vi "tes2-testModuleTurnsInvalidAPI.vi"(8 "error in (no error)":errorcluster, 11 "TestCase in":refnum<class "testcase-CSMNonCSMCallerSupportAPI.lvclass">) -> (0 "error out":errorcluster, 3 "TestCase out":refnum<class "testcase-CSMNonCSMCallerSupportAPI.lvclass">)   [LabVIEW 2017, in "testcase-CSMNonCSMCallerSupportAPI.lvclass"]
uses:
  testcase-CSMNonCSMCallerSupportAPI.lvclass
  <vilib>/addons/_JKI Toolkits/VI Tester/TestCase.llb/TestCase.lvclass
  src/user.lib/_NEVSTOP/Communicable State Machine(CSM)/Communicable State Machine.lvlib
  src/user.lib/_NEVSTOP/Communicable State Machine(CSM)/_Support/Typedef/_CSM_List Module Scope.ctl
  GlobalVariable_CSMModeData.vi
  InternalCluster.ctl
  C:/Program Files (x86)/National Instruments/LabVIEW 2017/vi.lib/addons/_JKI Toolkits/VI Tester/TestCase.llb/TestCase.lvclass
panel:
  in  "Stop":bool
  out "error out 2":errorcluster
  out "LoopCount":i32
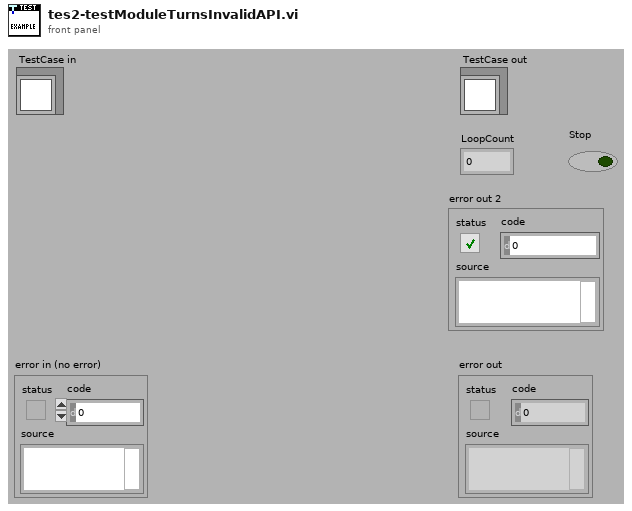
[diagram p1: front panel]
types:
  T1 = typedef "testcase-CSMNonCSMCallerSupportAPI.lvclass/InternalCluster.ctl" = cluster{"Mode":enum16{"Invalid", "Others", "WorkerAgent or Chain"}, "#Nodes":u32}
  T2 = typedef "Communicable State Machine.lvlib/_CSM_List Module Scope.ctl" = enum16{"Normal", "System Only", "All"}
  T3 = enum16{"Invalid", "Others", "WorkerAgent or Chain"}
  T4 = typedef "Communicable State Machine.lvlib/_CSM_MODE.ctl" = enum16{"Not Exist", "Stand Alone", "CSM", "Worker", "Worker Agent", "Chain Node", "Chain"}
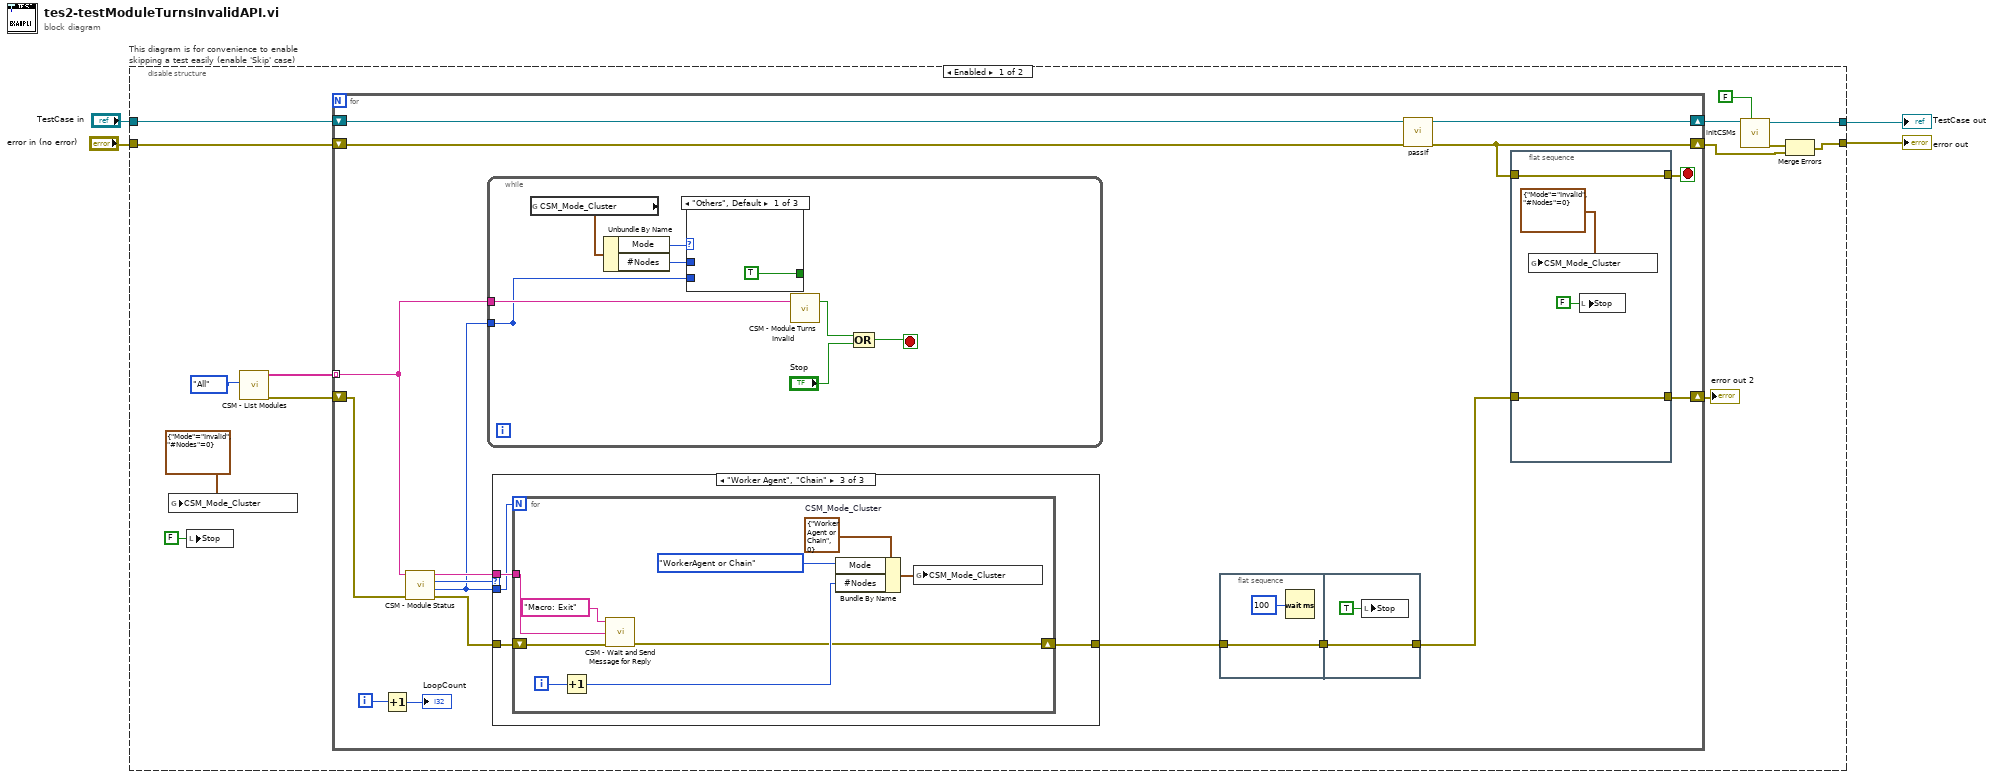
[diagram p0: block diagram]
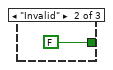
[diagram p2: hidden frame]
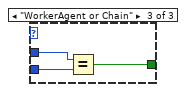
[diagram p3: hidden frame]
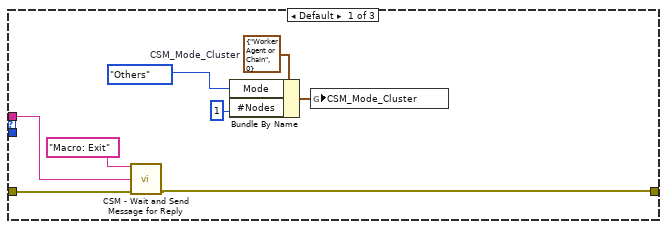
[diagram p4: hidden frame]
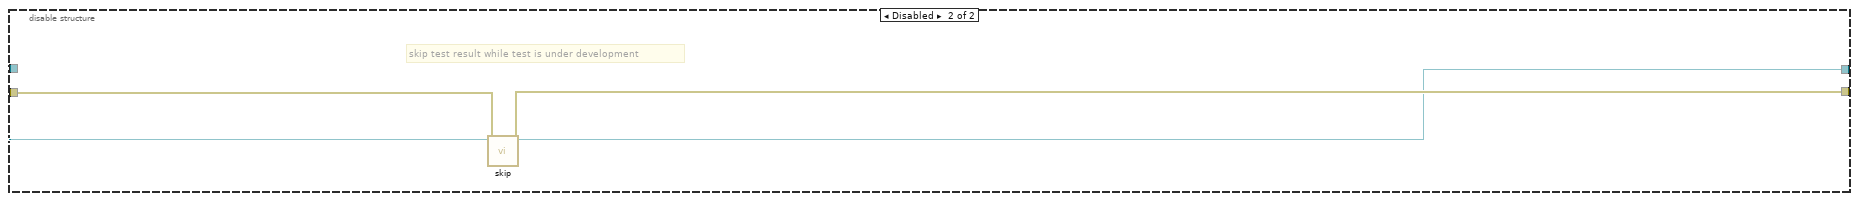
[diagram p6: hidden frame]
diagram:
  n1 = disable-structure "This diagram is for convenience to enable skipping a test easily (enable 'Skip' case)" shown="Enabled" {
    disable-tunnel: "TestCase in" -> [w16 w82]
    disable-tunnel: [w12 w80] -> w1
    disable-tunnel: [w9 w81] -> w3
    disable-tunnel: "error in (no error)" -> [w15 w79]
    frame Enabled {
      n2 = global write "GlobalVariable_CSMModeData.vi" "CSM_Mode_Cluster"(T1 {"Mode"=enum."Invalid", "#Nodes"=0} ("CSM_Mode_Cluster")) -> ()
      n3 = local write "Stop"(FALSE ("Stop")) -> ()
      n4 = call "CSM - List Modules.vi"("Scope (Normal)"=_CSM_List_Module_Scope."All") -> ("error out"=w17:errorcluster, "Module Names"=w6:string[])  [unwired: 9 in]
      n5 = for {
        shift-right: [w21] -> w8
        shift-left: w17 -> [w31]
        shift-right: [w26] -> w13
        shift-left: w16 -> [w33]
        shift-right: [w25] -> w10
        shift-left: w15 -> [w32]
        tunnel: w6 -> [w24] mode=indexing
        i -> [w35]
        stop <- w27 stop-if-true
        n6 = Increment(x=w35) -> (x+1=→"LoopCount":i32)
        n7 = call "CSM - Module Status.vi"("Error In"=w31, "CSM Name"=w24) -> ("error out"=w30:errorcluster, "#Nodes"=w19:i32, "Mode"=w29:T4, "CSM Name (Dup)"=w28:string)  [unwired: 5 in, 1 out]
        n8 = while {
          tunnel: w24 -> [w47]
          tunnel: [w40] -> _
          tunnel: w19 -> [w40]
          stop <- w45 stop-if-true
          n9 = global read "GlobalVariable_CSMModeData.vi" "CSM_Mode_Cluster"() -> (w43:T1)
          n10 = Unbundle By Name(w43) -> ("Mode"=w42:T3, "#Nodes"=w41:u32)
          n11 = case shown="\"Others\", Default" w42 {
            tunnel: [TRUE FALSE w51] -> _
            tunnel: w41 -> [_ _ w52]
            tunnel: w40 -> [_ _ w50]
            frame "Others", Default {
            }
            frame "Invalid" {
            }
            frame "WorkerAgent or Chain" {
              n12 = Equal?(x=w52, y=w50) -> (x = y?=w51:bool)
            }
          }
          n13 = call "CSM - Module Turns Invalid.vi"("CSM Name"=w47) -> ("Turn Invalid (Exit)?"=w44:bool)  [unwired: 2 in]
          n14 = Compound Arithmetic op=OR(w44, "Stop") -> (w45:bool)
        }
        n15 = case shown="\"Worker Agent\", \"Chain\"" w29 {
          tunnel: w30 -> [w64 w65 w69]
          tunnel: w19 -> [_ _ w67]
          tunnel: w28 -> [w62 _ w68]
          tunnel: [w57 w65 w66] -> w23
          frame Default {
            w61 = T1 {"Mode"=enum."WorkerAgent or Chain", "#Nodes"=0}  # CSM_Mode_Cluster
            n16 = call "CSM - Wait and Send Message for Reply.vi"("State"="Macro: Exit", "Target Module"=w62, "Error In (No Error)"=w64) -> ("error out"=w57:errorcluster)  [unwired: 10 in, 2 out]
            n17 = Bundle By Name(cluster=w61, "Mode"=T3."Others", "#Nodes"=u32 1) -> (w60:T1)
            n18 = global write "GlobalVariable_CSMModeData.vi" "CSM_Mode_Cluster"(w60) -> ()
          }
          frame "Not Exist" {
          }
          frame "Worker Agent", "Chain" {
            n19 = for {
              N: w67 -> [_]
              shift-right: [w70] -> w66
              shift-left: w69 -> [w78]
              tunnel: w68 -> [w75]
              i -> [w76]
              w74 = T1 {"Mode"=enum."WorkerAgent or Chain", "#Nodes"=0}  # CSM_Mode_Cluster
              n20 = Increment(x=w76) -> (x+1=w72:i32)
              n21 = call "CSM - Wait and Send Message for Reply.vi"("State"="Macro: Exit", "Target Module"=w75, "Error In (No Error)"=w78) -> ("error out"=w70:errorcluster)  [unwired: 10 in, 2 out]
              n22 = Bundle By Name(cluster=w74, "Mode"=T3."WorkerAgent or Chain", "#Nodes"=w72) -> (w73:T1)
              n23 = global write "GlobalVariable_CSMModeData.vi" "CSM_Mode_Cluster"(w73) -> ()
            }
          }
        }
        n24 = flat-sequence {
          tunnel: w23 -> [w37]
          tunnel: [w37] -> w22
          tunnel: [w39] -> w20
          tunnel: w22 -> [w39]
          frame #0 {
            n25 = Wait (ms)(milliseconds to wait=u32 100) -> ()  [unwired: 1 out]
          }
          frame #1 {
            n26 = local write "Stop"(TRUE ("Stop")) -> ()
          }
        }
        n27 = call-dynamic "passIf.vi"("error in (no error)"=w32, "TestCase in"=w33) -> ("error out"=w25:errorcluster, "TestCase out"=w26:refnum<class "testcase-CSMNonCSMCallerSupportAPI.lvclass">)  [unwired: 8 in]
        n28 = flat-sequence {
          tunnel: w25 -> [w55]
          tunnel: [w55] -> w27
          tunnel: [w53] -> w21
          tunnel: w20 -> [w53]
          frame #0 {
            n29 = global write "GlobalVariable_CSMModeData.vi" "CSM_Mode_Cluster"(T1 {"Mode"=enum."Invalid", "#Nodes"=0} ("CSM_Mode_Cluster")) -> ()
            n30 = local write "Stop"(FALSE ("Stop")) -> ()
          }
        }
      }
      "error out 2" <- w8
      n31 = call "initCSMs.vi"("Enable building lvlibp?"=FALSE, "TestCase in"=w13) -> ("error out"=w11:errorcluster, "TestCase out"=w12:refnum<class "testcase-CSMNonCSMCallerSupportAPI.lvclass">)  [unwired: 8 in]
      n32 = Merge Errors(w11, w10) -> (w9:errorcluster)
    }
    frame Disabled {
      # "skip test result while test is under development"
      n33 = call <vilib>:"skip.vi"("error in (no error)"=w79, "TestCase in"=w82) -> ("error out"=w81:errorcluster, "TestCase out"=w80:refnum<class "testcase-CSMNonCSMCallerSupportAPI.lvclass">)  [unwired: 8 in]
    }
  }
  "error out" <- w3
  "TestCase out" <- w1
